vi "get table.vi"(0 "db":dbl, 1 "pnColumn":i32, 5 "zSql":string, 7 "pazResult":string, 9 "pnRow":i32, 11 "error in (no error)":errorcluster, 12 "pzErrmsg":string) -> (3 "pnColumn out":i32, 4 "db out":dbl, 6 "function return":i32, 8 "pazResult out":string, 10 "pnRow out":i32, 14 "pzErrmsg out":string, 15 "error out":errorcluster)   [LabVIEW 2020, in "sqlite3.lvlib"]
uses:
  sqlite3.lvlib
  errstr.vi
  bin/sqlite3_64.dll
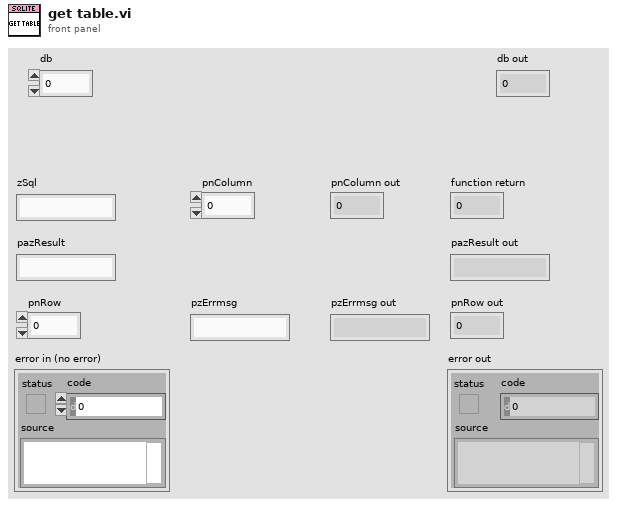
[diagram p1: front panel]
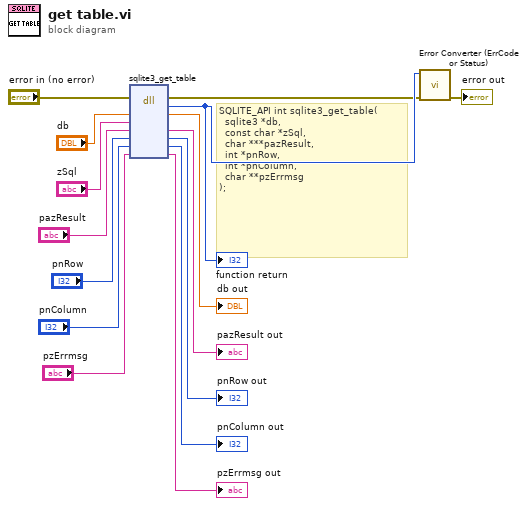
[diagram p0: block diagram]
diagram:
  # "SQLITE_API int sqlite3_get_table(\n  sqlite3 *db,          \n  const char *zSql,     \n  char ***pazResult,    \n  int *pnRow,           \n  int *pnColumn,        \n  char **pzErrmsg       \n);"
  n1 = dll-call lib="C:/Users/Fred.Guo/Desktop/Database-configuration/externals/sqlite3/Source/bin/sqlite3_*.*" fn="sqlite3_get_table"(error in="error in (no error)", "db"="db", "zSql"="zSql", "pazResult"="pazResult", "pnRow"="pnRow", "pnColumn"="pnColumn", "pzErrmsg"="pzErrmsg") -> (error out=w2:errorcluster, w15:i32, "db"=→"db out":dbl, "pazResult"=→"pazResult out":string, "pnRow"=→"pnRow out":i32, "pnColumn"=→"pnColumn out":i32, "pzErrmsg"=→"pzErrmsg out":string)  [unwired: 3 in, 1 out]
  "function return" <- w15
  n2 = call "Error Converter (ErrCode or Status).vi"("error in (no error)"=w2, "error code"=w15) -> ("error out"=→"error out":errorcluster)  [unwired: 9 in]
